vi "NewBlankExcelFile.vi"(8 "error in (no error)":errorcluster) -> (0 "error out":errorcluster, 3 "ExcelFile out":refnum<class "PortableExcelFileManipulationOXML.lvclass">)   [LabVIEW 2019, in "PortableExcelFileManipulationOXML.lvclass"]
doc: "Create a new excel file in memory with a spreadsheet named with the input string."
uses:
  PortableExcelFileManipulationOXML.lvclass
  H:/LV projects/ExpressionEvaluator/Excel/ExcelManipulation.dll
  ExcelManipulation.dll
  PortableExcelFileManipulationOXML.lvclass/PortableExcelFileManipulationOXML.ctl
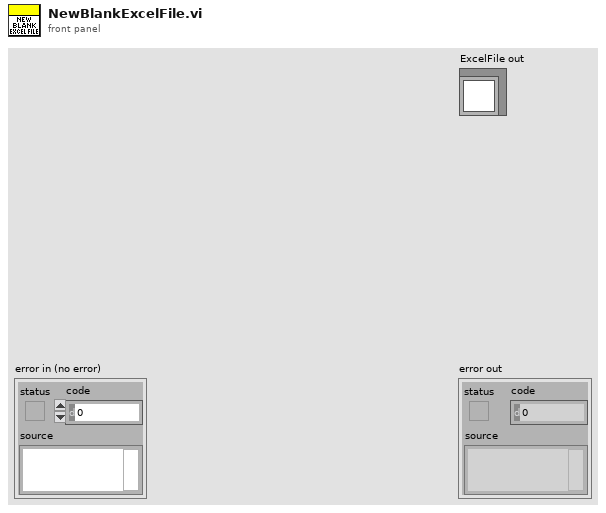
[diagram p1: front panel]
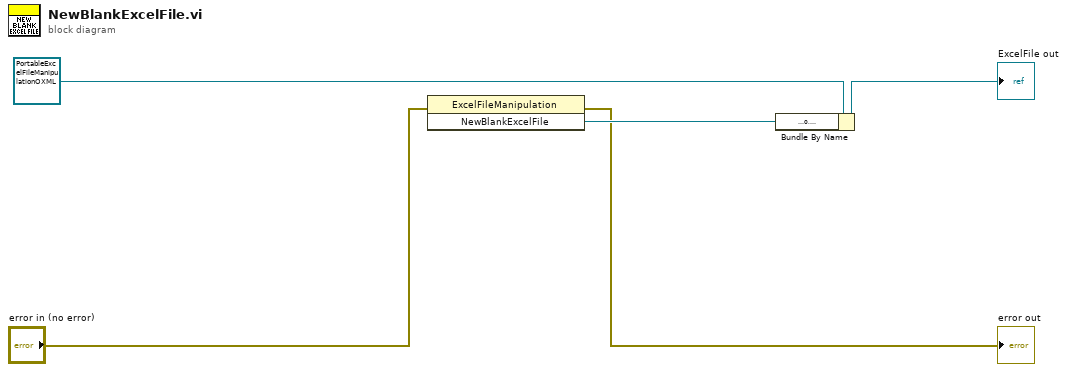
[diagram p0: block diagram]
diagram:
  n1 = invoke class="ExcelFileManipulation" method="NewBlankExcelFile"(error in="error in (no error)") -> (error out=→"error out":errorcluster, "NewBlankExcelFile"=w2:refnum<k24>)  [unwired: 2 in, 1 out]
  n2 = Bundle By Name(cluster=refnum<class "PortableExcelFileManipulationOXML.lvclass"> refnum ("ExcelFile in"), "ExcelOpen"=w2) -> (→"ExcelFile out":refnum<class "PortableExcelFileManipulationOXML.lvclass">)
